vi "SetSpeed_two_axis.vi"(2 "Acceleration Time 2":u16=100 max=1000, 3 "Acceleration Time 1":u16=100 max=1000, 4 "Port Number":i8=7 min=0, 5 "Low Speed 2":u32=100 min=1 max=500000, 6 "High Speed 2":u32=1000 min=1 max=500000, 7 "High Speed 1":u32=1000 min=1 max=500000, 8 "Low Speed 1":u32=100 min=1 max=500000) -> (0 "OK Done":bool, 1 "String Received":string)   [LabVIEW 2013]
panel:
  out "Command String":string
  # "Port Number 0=COM1"
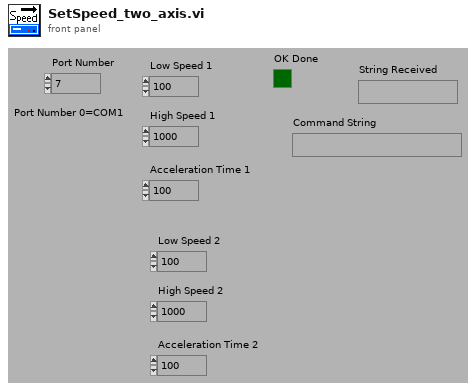
[diagram p1: front panel]
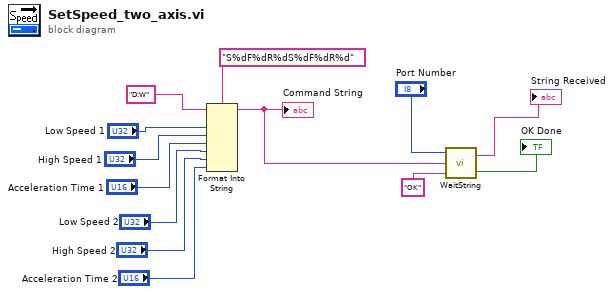
[diagram p0: block diagram]
diagram:
  n1 = Format Into String(format string="S%dF%dR%dS%dF%dR%d", initial string="D:W", "Low Speed 1", "High Speed 1", "Acceleration Time 1", "Low Speed 2", "High Speed 2", "Acceleration Time 2") -> (resulting string=w8:string)  [unwired: 1 in, 1 out]
  "Command String" <- w8
  n2 = call "WaitString.vi"("String to Receive"="OK", "String to Send"=w8, "PortNumber"="Port Number") -> ("OK Done"=→"OK Done":bool, "String Received"=→"String Received":string)
